vi "Gergberg Color.vi"() -> ()   [LabVIEW 2012, in "LightPipes.lvlib"]
uses:
  LightPipes.lvlib
panel:
  in  "Intensity Image Type":T1=2 items=["Grayscale (U8)", "Grayscale (I16)", "Grayscale (SGL)", "Complex (CSG)", "RGB (U32)", "HSL (U32)", "RGB (U64)", "Grayscale (U16)"]
  in  "Forward Distance":dbl(slide)=0.008365019011406844 step=0.0001 scale=-0.02..0.02
  in  "stop":bool
  out "Distance":dbl=0.008365019011406844
  out "Iteration":i32=49
  out "Original Far Field":T2(plugin-control)
  out "Original Mid Field":T2(plugin-control)
  out "error out":errorcluster
  in  "error in (no error)":errorcluster
  out "Far Field":T2(plugin-control)
  out "MF Phase":T2(plugin-control)
  out "Target Intensity\n RMS Error":dbl(graph)=324.4574427831586
  out "FF Phase":T2(plugin-control)
  out "Mid Field":T2(plugin-control)
  in  "n_grid":i32=250
  in  "lambda":dbl=1.054e-06
  in  "forward distance":dbl=0.02
  in  "size_grid":dbl=0.001776
  in  "Number of Iteration":i32=50
  in  "Far Field":path=path "E:/data4/FF Centered.png"
  in  "Mid Field":path=path "E:/data4/MF Centered.png"
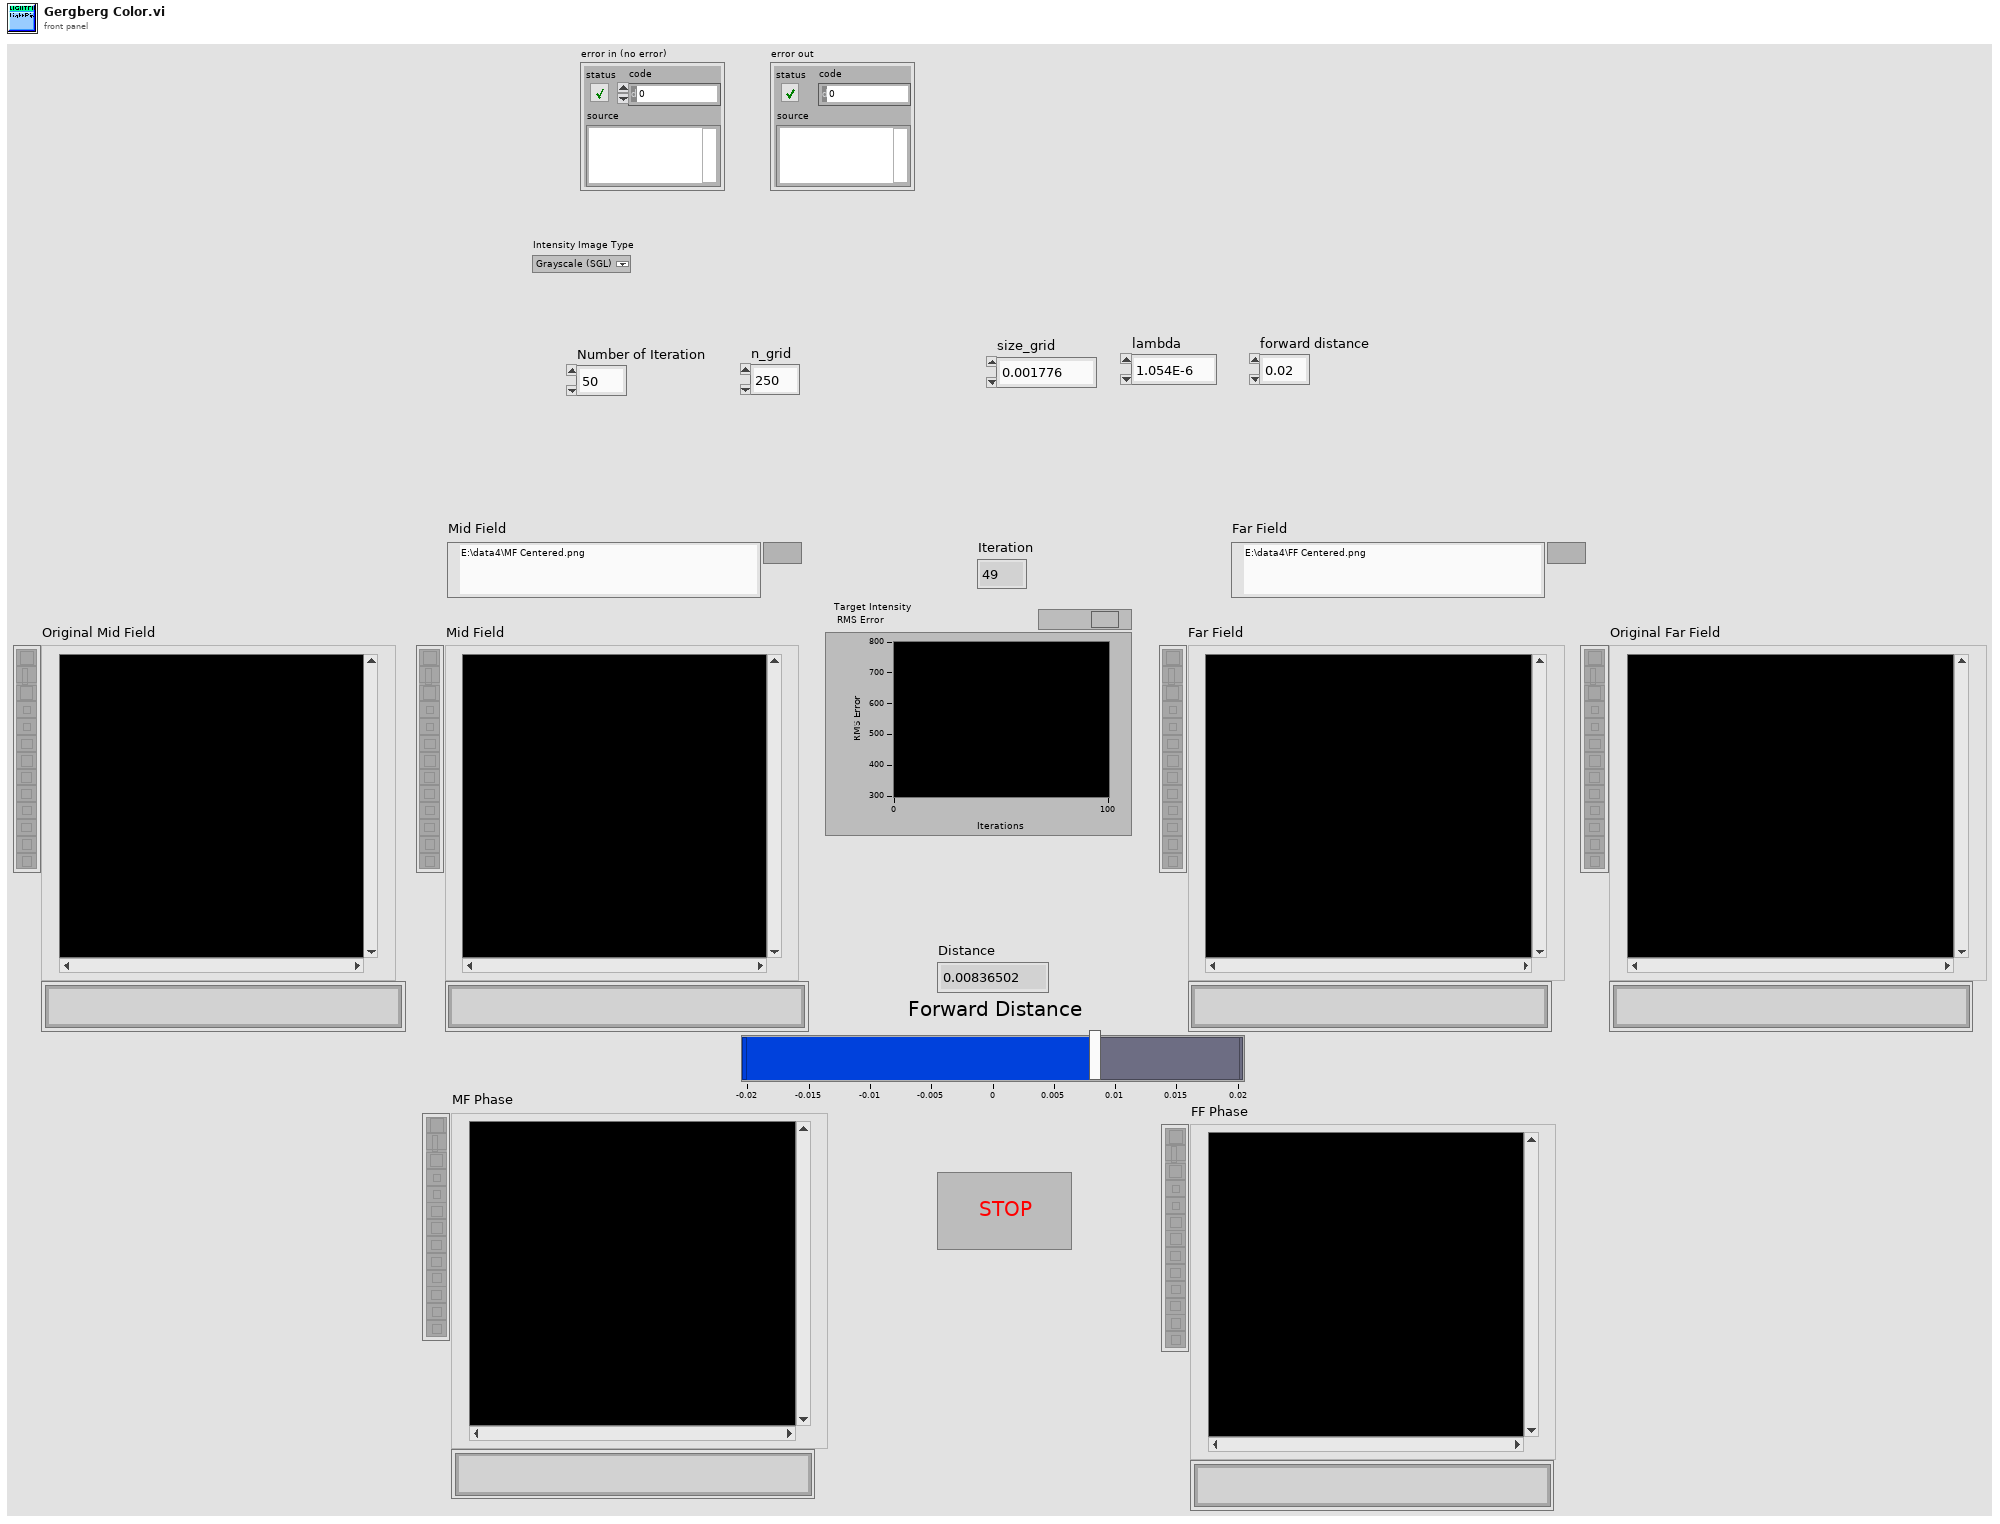
[diagram p1: front panel]
types:
  T1 = typedef "Image Type" = u32
  T2 = typedef "IMAQ Image.ctl" = refnum<image>
  T3 = cluster{"n_grid":i32, "@dummy control@":i8, "@dummy control@":i8, "@dummy control@":i8, "@dummy control@":i8, "size":dbl, "lambda":dbl, "int1":i32, "int2":i32, "int3":i32, "@dummy control@":i8, "@dummy control@":i8, "@dummy control@":i8, "@dummy control@":i8, "double1":dbl, "double2":dbl, "double3":dbl, "real":u32, "imaginary":u32}
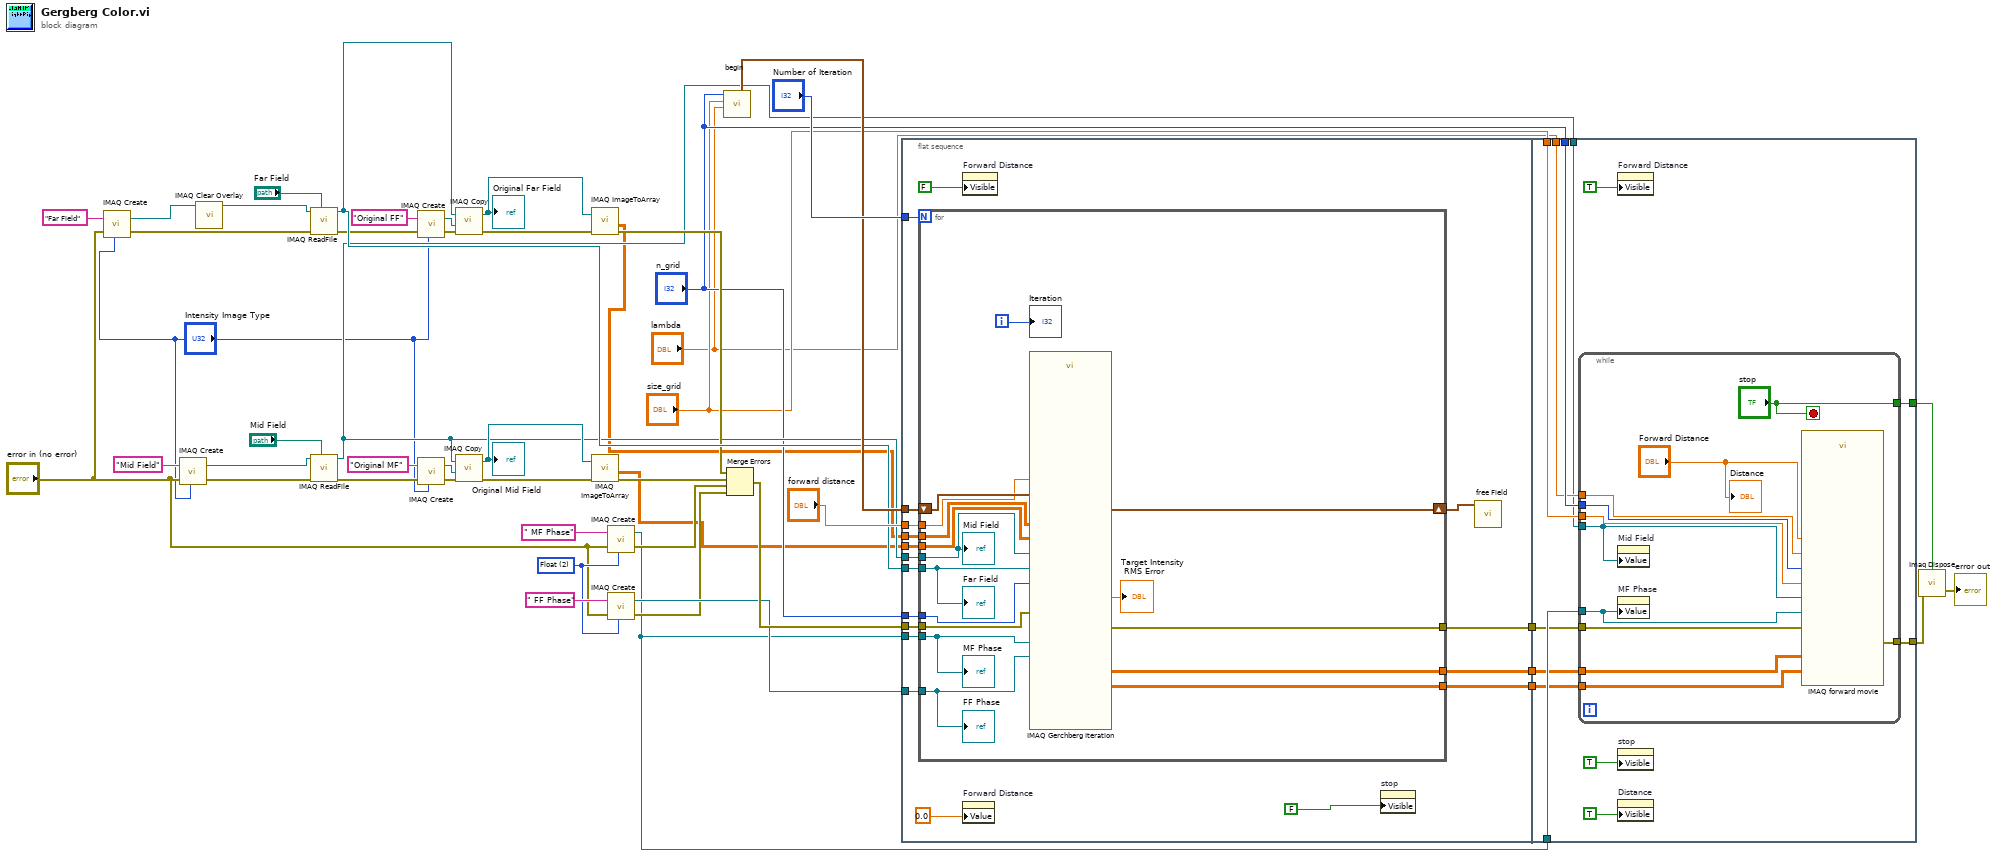
[diagram p0: block diagram]
diagram:
  w42 = u32 2 items=["8 bits", "16 bits", "Float", "Complex", "RGB", "HSL"] ("Image Type")
  n1 = call "IMAQ Create"("Image Name"="Far Field", "Image Type"="Intensity Image Type", "error in (no error)"="error in (no error)") -> ("New Image"=w17:T2, "error out"=w29:errorcluster)  [unwired: 2 in]
  n2 = call "IMAQ Create"("Image Name"="Mid Field", "Image Type"="Intensity Image Type", "error in (no error)"="error in (no error)") -> ("New Image"=w43:T2, "error out"=w27:errorcluster)  [unwired: 2 in]
  n3 = call "IMAQ Clear Overlay"("Image"=w17) -> ("Image Out"=w16:T2)  [unwired: 9 in, 1 out]
  n4 = call "IMAQ ReadFile"("File Path"="Far Field", "error in (no error)"=w29, "Image"=w16) -> ("error out"=w28:errorcluster, "Image Out"=w30:T2)  [unwired: 2 in, 5 out]
  n5 = call "IMAQ ReadFile"("File Path"="Mid Field", "error in (no error)"=w27, "Image"=w43) -> ("error out"=w26:errorcluster, "Image Out"=w10:T2)  [unwired: 2 in, 5 out]
  n6 = call "IMAQ Create"("Image Name"="Original FF", "Image Type"="Intensity Image Type", "error in (no error)"=w28) -> ("New Image"=w38:T2, "error out"=w37:errorcluster)  [unwired: 2 in]
  n7 = call "IMAQ Create"("Image Name"="Original MF", "Image Type"="Intensity Image Type", "error in (no error)"=w26) -> ("New Image"=w41:T2, "error out"=w40:errorcluster)  [unwired: 2 in]
  n8 = call "IMAQ Copy"("error in (no error)"=w37, "Image Dst"=w38, "Image Src"=w30) -> ("error out"=w32:errorcluster, "Image Dst Out"=w18:T2)  [unwired: 3 in]
  "Original Far Field" <- w18
  n9 = call "IMAQ Copy"("error in (no error)"=w40, "Image Dst"=w41, "Image Src"=w10) -> ("error out"=w31:errorcluster, "Image Dst Out"=w19:T2)  [unwired: 3 in]
  "Original Mid Field" <- w19
  n10 = call "IMAQ ImageToArray"("error in (no error)"=w32, "Image"=w18) -> ("Image Pixels (Float)"=w2:sgl[][], "error out"=w25:errorcluster)  [unwired: 2 in, 3 out]
  n11 = call "IMAQ ImageToArray"("error in (no error)"=w31, "Image"=w19) -> ("Image Pixels (Float)"=w1:sgl[][], "error out"=w24:errorcluster)  [unwired: 2 in, 3 out]
  n12 = call "IMAQ Create"("Image Name"=" MF Phase", "Image Type"=w42, "error in (no error)"="error in (no error)") -> ("New Image"=w11:T2, "error out"=w21:errorcluster)  [unwired: 2 in]
  n13 = call "IMAQ Create"("Image Name"=" FF Phase", "Image Type"=w42, "error in (no error)"="error in (no error)") -> ("New Image"=w22:T2, "error out"=w20:errorcluster)  [unwired: 2 in]
  n14 = call "begin.vi"("lambda"="lambda", "size_grid"="size_grid", "n_grid"="n_grid") -> ("field out"=w34:T3)  [unwired: 8 in]
  n15 = Merge Errors(w25, w24, w21, w20) -> (w23:errorcluster)
  n16 = flat-sequence {
    tunnel: "Number of Iteration" -> [w67]
    tunnel: w34 -> [w66]
    tunnel: "forward distance" -> [w65]
    tunnel: w10 -> [w63]
    tunnel: w30 -> [w62]
    tunnel: w23 -> [w61]
    tunnel: "n_grid" -> [w60]
    tunnel: w22 -> [w59]
    tunnel: w11 -> [w58]
    tunnel: w1 -> [w57]
    tunnel: w2 -> [w56]
    tunnel: [w55] -> w14
    tunnel: [w52] -> w5
    tunnel: [w51] -> w4
    tunnel: w14 -> [w84]
    tunnel: [w95] -> w12
    tunnel: w11 -> [w87]
    tunnel: w10 -> [w88]
    tunnel: "n_grid" -> [w94]
    tunnel: "size_grid" -> [w93]
    tunnel: "lambda" -> [w92]
    tunnel: [w91] -> w6
    tunnel: w5 -> [w86]
    tunnel: w4 -> [w85]
    frame #0 {
      n17 = for {
        N: w67 -> [_]
        shift-right: [w82] -> w64
        shift-left: w66 -> [w83]
        tunnel: w65 -> [w81]
        tunnel: w57 -> [w69]
        tunnel: w56 -> [w77]
        tunnel: w63 -> [w75]
        tunnel: w62 -> [w74]
        tunnel: w61 -> [w80]
        tunnel: [w79] -> w55
        tunnel: w60 -> [w78]
        tunnel: w59 -> [w71]
        tunnel: w58 -> [w72]
        tunnel: [w68] -> w52
        tunnel: [w70] -> w51
        i -> [w76]
        n18 = call "IMAQ Gerchberg Iteration.vi"("field"=w83, "Original Source"=w69, "n_grid"=w78, "forward distance"=w81, "Original Target"=w77, "error in (no error)"=w80, "Source"=w75, "Target"=w74, "Source Phase"=w72, "Target Phase"=w71) -> ("Source Intensity"=w68:dbl[][], "Source Phase"=w70:dbl[][], "field out"=w82:T3, "Target Intensity\n RMS Error"=→"Target Intensity\n RMS Error":dbl, "error out"=w79:errorcluster)  [unwired: 3 in, 2 out]
        "Iteration" <- w76
        "Mid Field" <- w75
        "Far Field" <- w74
        "MF Phase" <- w72
        "FF Phase" <- w71
      }
      n19 = property on="Forward Distance" class="Slide (strict)"("Visible"=FALSE) -> ()  [unwired: 2 in, 2 out]
      n20 = property on="Forward Distance" class="Slide (strict)"("Value"=0.0 ("Forward Distance")) -> ()  [unwired: 2 in, 2 out]
      n21 = property on="stop" class="Bool"("Visible"=FALSE) -> ()  [unwired: 2 in, 2 out]
      n22 = call "free Field.vi"("field"=w64) -> ()  [unwired: 10 in, 1 out]
    }
    frame #1 {
      n23 = while {
        tunnel: ["stop"] -> w95
        tunnel: w87 -> [w98]
        tunnel: w88 -> [w99]
        tunnel: w94 -> [w106]
        tunnel: w93 -> [w105]
        tunnel: w92 -> [w104]
        tunnel: [w101] -> w91
        tunnel: w84 -> [w102]
        tunnel: w86 -> [w97]
        tunnel: w85 -> [w100]
        stop <- "stop" stop-if-true
        n24 = property on="Mid Field" class="ImageControl"("Value"=w99) -> ()  [unwired: 2 in, 2 out]
        n25 = property on="MF Phase" class="ImageControl"("Value"=w98) -> ()  [unwired: 2 in, 2 out]
        n26 = call "IMAQ forward movie.vi"("Forwarded Phase"=w98, "n_grid"=w106, "Source Intensity"=w97, "Forwarded Intensity"=w99, "error in (no error)"=w102, "size_grid"=w105, "lambda"=w104, "Forward Distance"="Forward Distance", "Source Phase"=w100) -> ("error out"=w101:errorcluster)  [unwired: 6 in]
        "Distance" <- "Forward Distance"
      }
      n27 = property on="Forward Distance" class="Slide (strict)"("Visible"=TRUE) -> ()  [unwired: 2 in, 2 out]
      n28 = property on="stop" class="Bool"("Visible"=TRUE) -> ()  [unwired: 2 in, 2 out]
      n29 = property on="Distance" class="DigNum (strict)"("Visible"=TRUE) -> ()  [unwired: 2 in, 2 out]
    }
  }
  n30 = call "Imaq Dispose"("All Images? (No)"=w12, "error in (no error)"=w6) -> ("error out"=→"error out":errorcluster)  [unwired: 4 in]
